vi "CP_Launch.vi"(0 "SubPanel Ref":refnum<vi>, 5 "vi reference":refnum<vi>, 7 "Control Init Array":T1(array[cluster]), 9 "Window Title (opt)":string, 11 "error in (no error)":errorcluster) -> (15 "error out":errorcluster)   [LabVIEW 2009]
doc: "Part of the Dock/Undock demonstration of Sub Panels. Contributed by www.entzen.com.\n\nAAL 9/09"
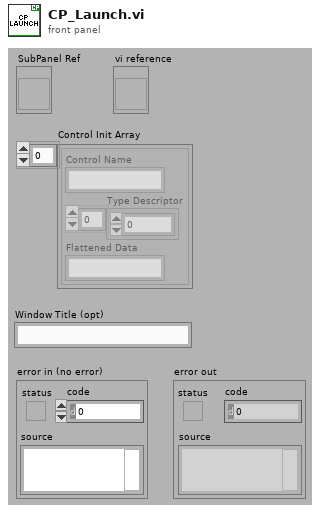
[diagram p1: front panel]
types:
  T1 = cluster{"Control Name":string, "Type Descriptor":i16[], "Flattened Data":string}[]
  T2 = typedef "LVRectTypeDef.ctl" = cluster{"left":i16, "top":i16, "right":i16, "bottom":i16}
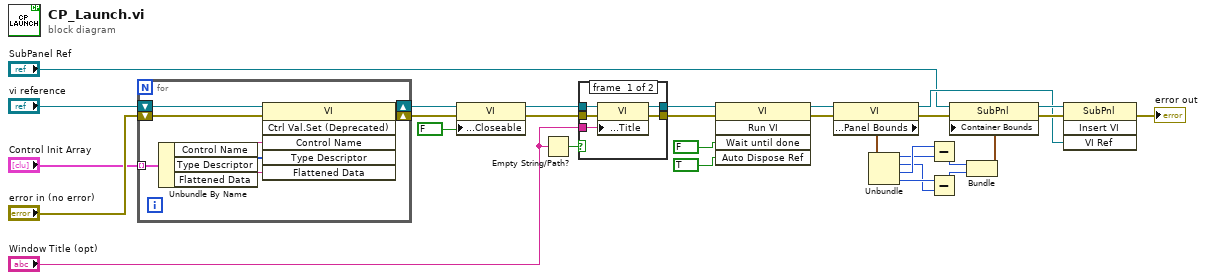
[diagram p0: block diagram]
diagram:
  n1 = for {
    shift-right: [w37] -> w8
    shift-left: "error in (no error)" -> [w35]
    shift-right: [w38] -> w9
    shift-left: "vi reference" -> [w36]
    tunnel: "Control Init Array" -> [w34] mode=indexing
    n2 = Unbundle By Name(w34) -> ("Control Name"=w33:string, "Type Descriptor"=w32:i16[], "Flattened Data"=w31:string)
    n3 = invoke class="VI" method="Ctrl Val.Set (Deprecated)"(reference=w36, error in=w35, "Control Name"=w33, "Type Descriptor"=w32, "Flattened Data"=w31) -> (reference out=w38:refnum<vi>, error out=w37:errorcluster)  [unwired: 1 in, 4 out]
  }
  n4 = property class="VI"(reference=w9, error in=w8, "Front Panel Window:Closeable"=FALSE) -> (reference out=w6:refnum<vi>, error out=w5:errorcluster)
  n5 = Empty String/Path?(string/path="Window Title (opt)") -> (empty?=w1:bool)
  n6 = case shown="False" w1 {
    tunnel: "Window Title (opt)" -> [w43 _]
    tunnel: w6 -> [w42 w45]
    tunnel: w5 -> [w41 w44]
    tunnel: [w40 w44] -> w4
    tunnel: [w39 w45] -> w3
    frame #0 {
      n7 = property class="VI"(reference=w42, error in=w41, "Front Panel Window:Title"=w43) -> (reference out=w39:refnum<vi>, error out=w40:errorcluster)
    }
    frame #1 {
    }
  }
  n8 = invoke class="VI" method="Run VI"(reference=w3, error in=w4, "Wait until done"=FALSE, "Auto Dispose Ref"=TRUE) -> (reference out=w19:refnum<vi>, error out=w18:errorcluster)  [unwired: 1 in, 3 out]
  n9 = property on="Property Node" class="VI"(reference=w19, error in=w18) -> (reference out=w14:refnum<vi>, error out=w15:errorcluster, "Front Panel Window:Panel Bounds"=w29:T2)
  n10 = Unbundle(w29) -> ("left"=w27:i16, "top"=w25:i16, "right"=w28:i16, "bottom"=w26:i16)
  n11 = Subtract(x=w28, y=w27) -> (x-y=w24:i16)
  n12 = Subtract(x=w26, y=w25) -> (x-y=w23:i16)
  n13 = Bundle(w24, w23) -> (w22:cluster{i16, i16})  [unwired: 1 in]
  n14 = property on="Property Node" class="SubPnl"(reference="SubPanel Ref", error in=w15, "Container Bounds"=w22) -> (reference out=w17:refnum<vi>, error out=w16:errorcluster)
  n15 = invoke on="Invoke Node" class="SubPnl" method="Insert VI"(reference=w17, error in=w16, "VI Ref"=w14) -> (error out=→"error out":errorcluster)  [unwired: 1 in, 3 out]
